vi "Init.vi"(8 "error in (no error)":errorcluster, 11 "VISA resource name":refnum<visa-resource-name>) -> (0 "error out":errorcluster, 3 "VISA resource name out":refnum<visa-resource-name>)   [LabVIEW 2024, in "Revidyne Generator.lvlib"]
doc: "This vi will cause the generator to spin up and then stop."
uses:
  Revidyne Generator.lvlib
  2445cd8c-2b24-46d9-a207-312452237bbc.vi
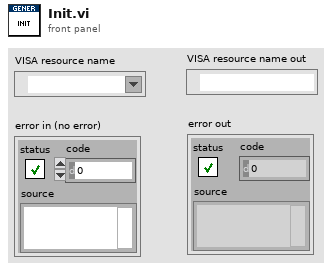
[diagram p1: front panel]
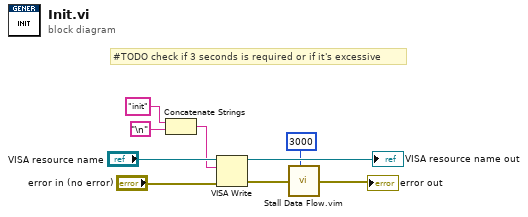
[diagram p0: block diagram]
diagram:
  # "#TODO check if 3 seconds is required or if it's excessive"
  n1 = Concatenate Strings("init" ("command"), "\n") -> (w2:string)
  n2 = VISA Write(VISA resource name="VISA resource name", write buffer=w2, error in (no error)="error in (no error)") -> (VISA resource name out=→"VISA resource name out":refnum<visa-resource-name>, error out=w6:errorcluster)  [unwired: 1 out]
  n3 = call "Stall Data Flow.vim"("value in"=w6, "milliseconds to wait"=u32 3000) -> ("value out"=→"error out":errorcluster)  [unwired: 1 out]
